vi "List Available Printers.vi"(8 "error in (no error)":errorcluster) -> (0 "error out":errorcluster, 2 "Default Printer":string, 3 "Available Printers":string[](array[string]))   [LabVIEW 2017]
uses:
  <userlib>/_OpenG.lib/array/array.llb/Filter 1D Array (String)__ogtk.vi
  <userlib>/_OpenG.lib/string/string.llb/Trim Whitespace (String Array)__ogtk.vi
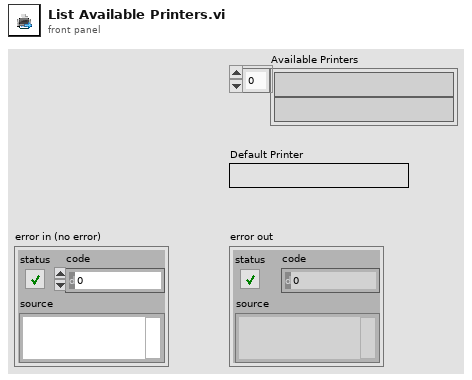
[diagram p1: front panel]
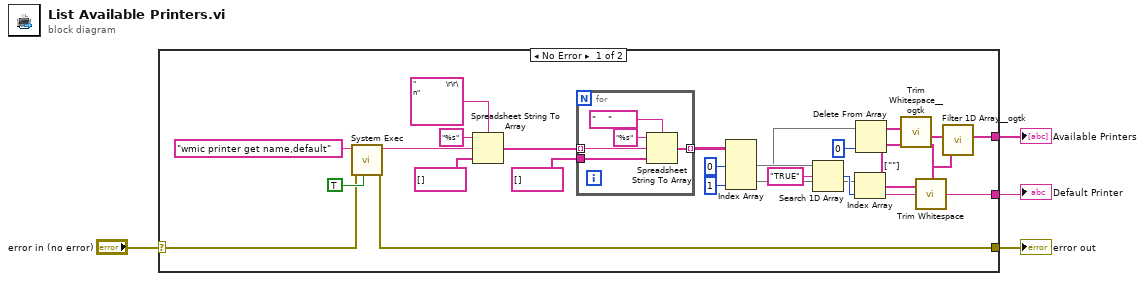
[diagram p0: block diagram]
diagram:
  n1 = case shown="No Error" "error in (no error)" {
    selector: "error in (no error)" -> [w10 w34]
    tunnel: [w5 _] -> w4
    tunnel: [w7 _] -> w3
    tunnel: [w11 w34] -> w2
    frame No Error {
      n2 = call <vilib>:"System Exec.vi"("run minimized? (F)"=TRUE, "error in (no error)"=w10, "command line"="wmic printer get name,default") -> ("error out"=w11:errorcluster, "standard output"=w27:string)  [unwired: 5 in, 2 out]
      n3 = Spreadsheet String To Array(delimiter (Tab)="               \r\r\n", format string="%s", spreadsheet string=w27, array type (2D Dbl)=string[] [] ("format string")) -> (array=w23:string[])
      n4 = for {
        tunnel: w23 -> [w33] mode=indexing
        tunnel: string[] [] ("format string") -> [w32]
        tunnel: [w29] -> w22 mode=indexing
        n5 = Spreadsheet String To Array(delimiter (Tab)="    ", format string="%s", spreadsheet string=w33, array type (2D Dbl)=w32) -> (array=w29:string[])
      }
      n6 = Index Array(array=w22, index (col) #1=0 ("disabled index (col)"), index (col) #2=1 ("disabled index (col)")) -> (element #1=w21:string[], element #2=w13:string[])  [unwired: 2 in]
      n7 = Search 1D Array(1D array=w21, element="TRUE") -> (index of element=w18:i32)  [unwired: 1 in]
      n8 = Index Array(array=w13, index=w18) -> (element=w17:string)
      n9 = Delete From Array(array=w13, index=0) -> (array with subset deleted=w9:string[])  [unwired: 1 in, 1 out]
      n10 = call-poly <userlib>:"Trim Whitespace__ogtk.vi"("String in"=w9) -> ("String out"=w8:string[])  [unwired: 6 in]
      n11 = call <vilib>:"Trim Whitespace.vi"("string"=w17) -> ("trimmed string"=w5:string)  [unwired: 1 in]
      n12 = call-poly <userlib>:"Filter 1D Array__ogtk.vi"("items to filter"=string[] [""], "array"=w8) -> ("filtered array"=w7:string[])  [unwired: 4 in, 1 out]
    }
    frame Error {
    }
  }
  "Default Printer" <- w4
  "Available Printers" <- w3
  "error out" <- w2
